vi "Test-Fpga-CryptoNight-Step-3.vi"() -> ()   [LabVIEW 2017]
panel:
  out "hp_state out (FPGA)":u64[](array[numeric]) format="%.0x"
  out "Values Match?":bool
  out "exp_hp_state_out":u64[](array[numeric]) format="%.0x"
  out "Runtime (minutes)":dbl
  in  "Override Iterations":bool=TRUE
  out "Runtime (s)":dbl
  out "Runtime (ms)":u32
  in  "# of Iterations":i32
  out "hp_state out":u64[](array[numeric]) format="%.0x"
  out "b_out":u64[](array[numeric]) format="%.0x"
  out "a_out":u64[](array[numeric]) format="%.0x"
  in  "FileName":string="log_file.8.bin"
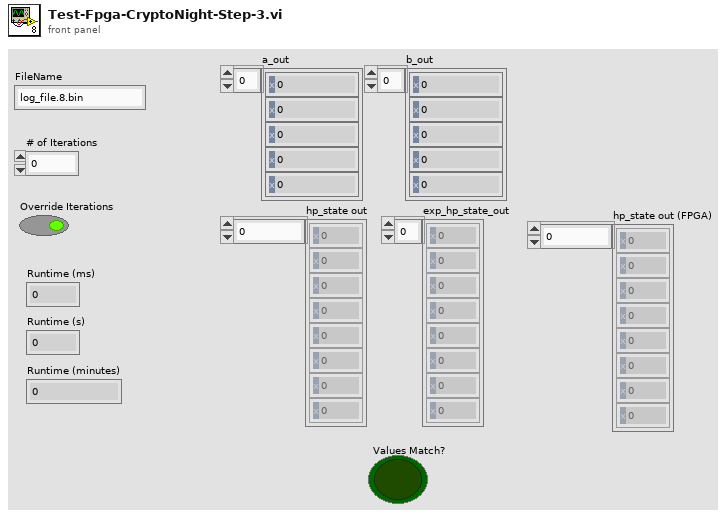
[diagram p1: front panel]
types:
  T1 = typedef "Step-3-Data-Type.ctl" = cluster{"a":u64[], "b":u64[], "hp_state_in":u8[], "hp_state_out":u8[], "hp_state_in (u64)":u64[], "hp_state_out (u64)":u64[]}
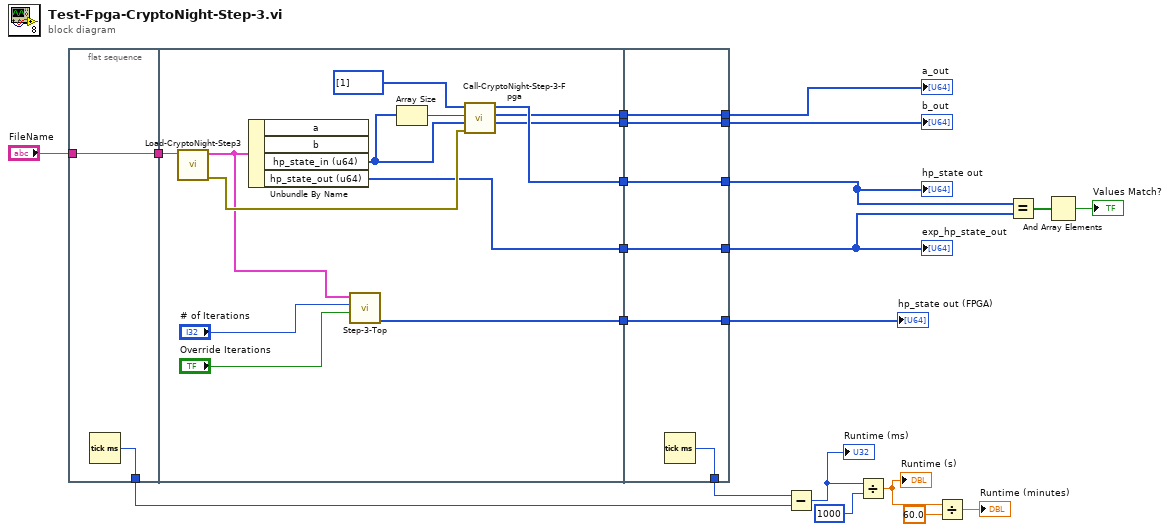
[diagram p0: block diagram]
diagram:
  n1 = flat-sequence {
    tunnel: "FileName" -> [w23]
    tunnel: [w23] -> w17
    tunnel: [w22] -> w15
    tunnel: [w30] -> w18
    tunnel: w17 -> [w36]
    tunnel: [w31] -> w7
    tunnel: [w29] -> w6
    tunnel: [w28] -> w3
    tunnel: [w24] -> w1
    tunnel: [w41] -> w19
    tunnel: [w42] -> w20
    tunnel: w18 -> [w42]
    tunnel: [w40] -> w16
    tunnel: [w39] -> w5
    tunnel: w7 -> [w39]
    tunnel: w6 -> [w41]
    tunnel: [w38] -> w4
    tunnel: w3 -> [w38]
    tunnel: [w37] -> w2
    tunnel: w1 -> [w37]
    frame #0 {
      n2 = Tick Count (ms)() -> (millisecond timer value=w22:u32)
    }
    frame #1 {
      n3 = call "Load-CryptoNight-Step3.vi"("FileName"=w36) -> ("error out"=w32:errorcluster, "output cluster"=w27:T1)  [unwired: 9 in]
      n4 = Unbundle By Name(w27) -> ("hp_state_in (u64)"=w34:u64[], "hp_state_out (u64)"=w28:u64[])  [unwired: 2 out]
      n5 = call "Step-3-Top.vi"("Override Iterations"="Override Iterations", "# of Iterations"="# of Iterations", "input"=w27) -> ("hp_state out (u64)"=w24:u64[])  [unwired: 6 in, 2 out]
      n6 = Array Size(array=w34) -> (size(s)=w33:i32)
      n7 = call "Call-CryptoNight-Step-3-Fpga.vi"("error in"=w32, "Data in"=w34, "Size-in"=w33, "Command"=u32[] [1]) -> ("b_out"=w29:u64[], "a_out"=w30:u64[], "Data out"=w31:u64[])  [unwired: 4 in, 1 out]
    }
    frame #2 {
      n8 = Tick Count (ms)() -> (millisecond timer value=w40:u32)
    }
  }
  n9 = Subtract(x=w16, y=w15) -> (x-y=w14:u32)
  "Runtime (ms)" <- w14
  n10 = Divide(x=w14, y=u32 1000) -> (x/y=w12:dbl)
  "Runtime (s)" <- w12
  n11 = Divide(x=w12, y=60.0) -> (x/y=→"Runtime (minutes)":dbl)
  n12 = Equal?(x=w5, y=w4) -> (x = y?=w9:bool[])
  n13 = And Array Elements(Boolean array=w9) -> (logical AND=→"Values Match?":bool)
  "a_out" <- w20
  "b_out" <- w19
  "hp_state out" <- w5
  "exp_hp_state_out" <- w4
  "hp_state out (FPGA)" <- w2
